vi "Stop Core.vi"(10 "final error code":i32, 11 "NI in":refnum<class "NI.lvclass">) -> (3 "NI out":refnum<class "NI.lvclass">)   [LabVIEW 2021, in "NI.lvlib" / "NI.lvclass"]
doc: "(<B>Filename</B>: Actor Framework.lvlib:Actor.lvclass:Stop Core.vi)\n\nDefines what the actor does before it stops. Use the <B>final error code</B> input to determine whether the actor shut down in response to an error.\n\nBy default, this method does nothing. A descendant class may override it to define behavior, such as shutting down any processes the actor initiated in its override of the Actor Core method."
uses:
  NI.lvclass
  Channel Connection.ctl
  NI.lvclass/NI.ctl
  Utilities/RWC_Actions.ctl
  <vilib>/ActorFramework/Actor/Actor.lvclass
panel:
  out "error out":errorcluster
  out "Inner parameters":T2
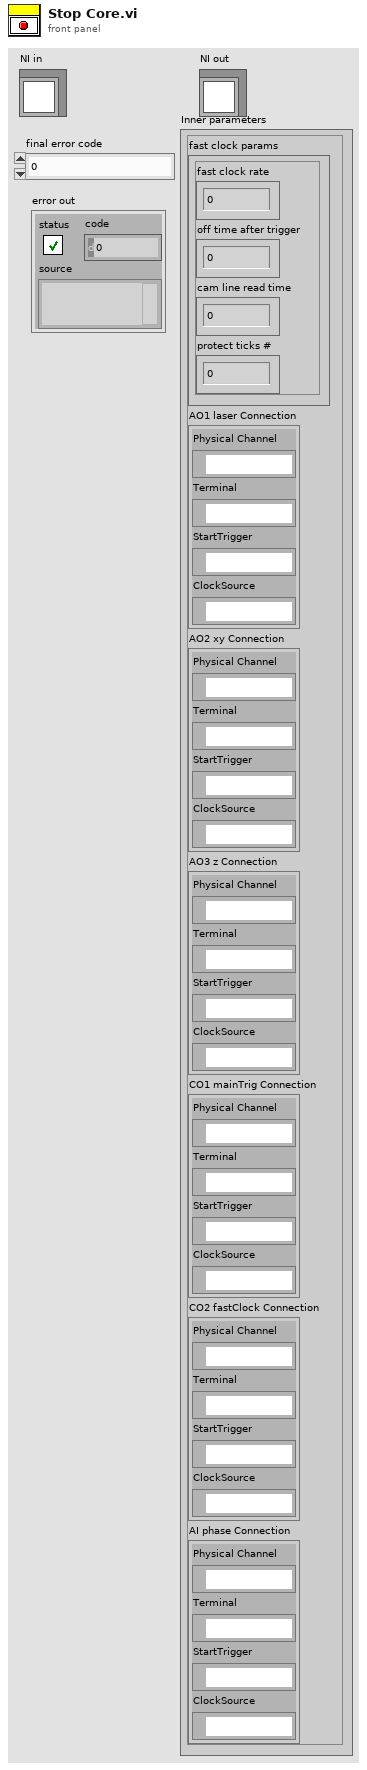
[diagram p1: front panel]
types:
  T1 = typedef "NI.lvlib/NI.lvclass/Channel Connection.ctl" = cluster{"Physical Channel":tag, "Terminal":tag, "StartTrigger":tag, "ClockSource":tag}
  T2 = cluster{"fast clock params":cluster{"fast clock rate":dbl, "off time after trigger":dbl, "cam line read time":dbl, "protect ticks #":dbl}, "AO1 laser Connection":T1, "AO2 xy Connection":T1, "AO3 z Connection":T1, "CO1 mainTrig Connection":T1, "CO2 fastClock Connection":T1, "AI phase Connection":T1}
  T3 = cluster{"fast clock params":cluster{"fast clock rate":dbl, "off time after trigger":dbl, "cam line read time":dbl, "protect ticks #":dbl}, "AO1 laser Connection":T1, "AO2 zy Connection":T1, "AO3 z Connection (deprecated)":T1, "CO1 mainTrig Connection":T1, "CO2 fastClock Connection":T1, "AI phase Connection":T1}
  T4 = typedef "RWC_Actions.ctl" = enum16{"Read", "Write", "Read and Create"}
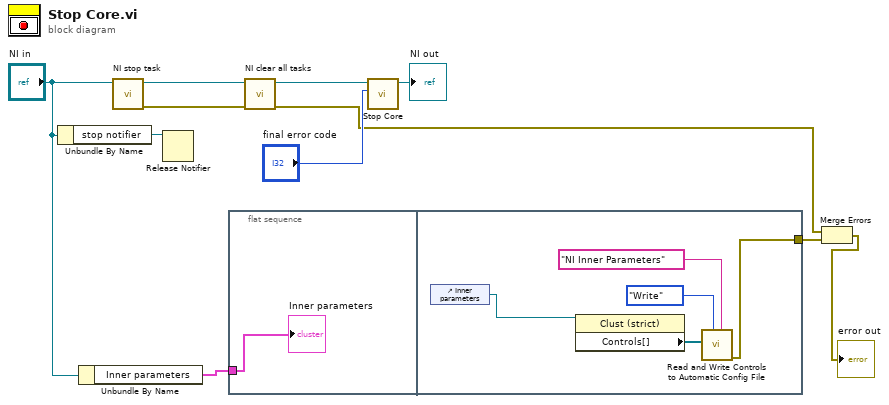
[diagram p0: block diagram]
diagram:
  n1 = Unbundle By Name("NI in") -> ("stop notifier"=w9:refnum<notifier>)
  n2 = Unbundle By Name("NI in") -> ("Inner parameters"=w5:T3)
  n3 = call "NI stop task.vi"("NI in"="NI in") -> ("error out"=w4:errorcluster, "NI out"=w8:refnum<class "NI.lvclass">)  [unwired: 9 in]
  n4 = Release Notifier(notifier=w9) -> ()  [unwired: 2 in, 3 out]
  n5 = flat-sequence {
    tunnel: w5 -> [w12]
    tunnel: [w13] -> w2
    frame #0 {
      "Inner parameters" <- w12
    }
    frame #1 {
      n6 = control-ref of="Inner parameters"() -> (w14:refnum<vi>)
      n7 = property class="Clust (strict)"(reference=w14) -> ("Controls[]"=w15:refnum<vi>[])  [unwired: 1 in, 2 out]
      n8 = call "Read and Write Controls to Automatic Config File.vi"("file name"="NI Inner Parameters" ("section (optional)"), "Action"=RWC_Actions."Write", "Control References"=w15) -> ("error out"=w13:errorcluster)  [unwired: 8 in]
    }
  }
  n9 = call "NI clear all tasks.vi"("error in (no error)"=w4, "NI in"=w8) -> ("error out"=w3:errorcluster, "NI out"=w7:refnum<class "NI.lvclass">)  [unwired: 8 in]
  n10 = call-parent "Stop Core.vi"("final error code"="final error code", "Actor in"=w7) -> ("Actor out"=→"NI out":refnum<class "NI.lvclass">)  [unwired: 9 in]
  n11 = Merge Errors(w3, w2) -> (→"error out":errorcluster)
